vi "Bump Version.vi"(4 "Version Type":T2=enum."Fix", 5 "Previous Version":T1, 6 "Increment Build (T)":bool=TRUE) -> (7 "Next Version":T1)   [LabVIEW 2020, in "Builder Core.lvlib"]
uses:
  Builder Core.lvlib
  Version.ctl
  Version Type.ctl
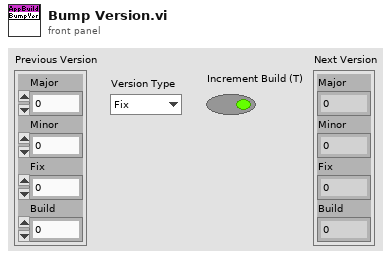
[diagram p1: front panel]
types:
  T1 = typedef "Builder Core.lvlib/Version.ctl" = cluster{"Major":u16, "Minor":u16, "Fix":u16, "Build":u16}
  T2 = typedef "Builder Core.lvlib/Version Type.ctl" = enum16{"None", "Fix", "Minor", "Major"}
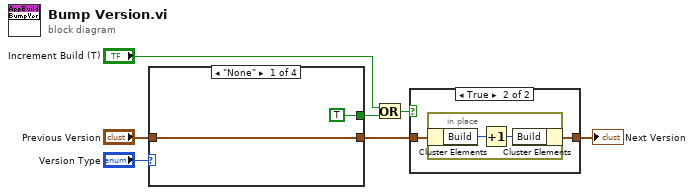
[diagram p0: block diagram]
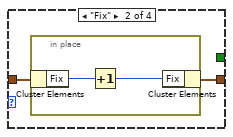
[diagram p3: hidden frame]
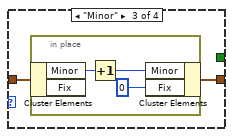
[diagram p4: hidden frame]
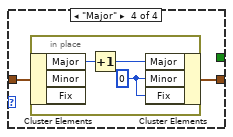
[diagram p5: hidden frame]
diagram:
  n1 = case shown="\"None\"" "Version Type" {
    tunnel: "Previous Version" -> [w8 w11 w15 w20]
    tunnel: [TRUE _ _ _] -> w5
    tunnel: [w8 w10 w14 w19] -> w3
    frame "None" {
    }
    frame "Fix" {
      n2 = in-place {
        n3 = in-place-cluster #1(w11) -> ("Fix"=w13:u16)
        n4 = Increment(x=w13) -> (x+1=w12:u16)
        n5 = in-place-cluster #1("Fix"=w12) -> (w10:T1)
      }
    }
    frame "Minor" {
      n6 = in-place {
        n7 = in-place-cluster #2(w15) -> ("Minor"=w17:u16)  [unwired: 1 out]
        n8 = Increment(x=w17) -> (x+1=w16:u16)
        n9 = in-place-cluster #2("Minor"=w16, "Fix"=u16 0 ("Minor")) -> (w14:T1)
      }
    }
    frame "Major" {
      n10 = in-place {
        w23 = u16 0 ("Minor")
        n11 = in-place-cluster #3(w20) -> ("Major"=w22:u16)  [unwired: 2 out]
        n12 = Increment(x=w22) -> (x+1=w21:u16)
        n13 = in-place-cluster #3("Major"=w21, "Minor"=w23, "Fix"=w23) -> (w19:T1)
      }
    }
  }
  n14 = Or(x="Increment Build (T)", y=w5) -> (x .or. y?=w2:bool)
  n15 = case shown="True" w2 {
    tunnel: w3 -> [w24 w26]
    tunnel: [w24 w25] -> w1
    frame False {
    }
    frame True {
      n16 = in-place {
        n17 = in-place-cluster #4(w26) -> ("Build"=w28:u16)
        n18 = Increment(x=w28) -> (x+1=w27:u16)
        n19 = in-place-cluster #4("Build"=w27) -> (w25:T1)
      }
    }
  }
  "Next Version" <- w1
